vi "экзамен  (SubVI).vi"(6 "N":i32(slide) scale=0.0..10.0, 9 "C":dbl(slide) scale=0.0..10.0, 10 "B":dbl(slide) scale=0.0..10.0, 11 "A":dbl(slide) scale=0.0..10.0) -> ()   [LabVIEW 2012]
panel:
  out "Waveform Graph":dbl[](graph)
  out "Boolean":bool
  out "DC":dbl format="%#_3g"
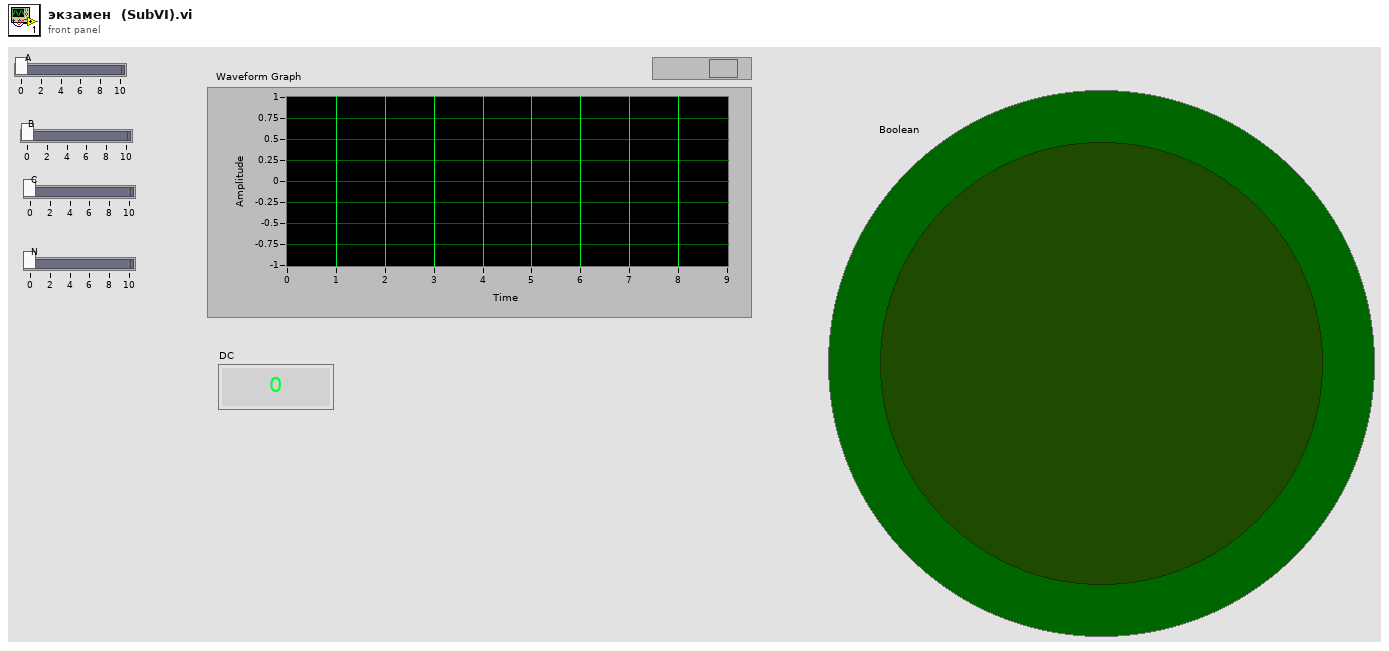
[diagram p1: front panel]
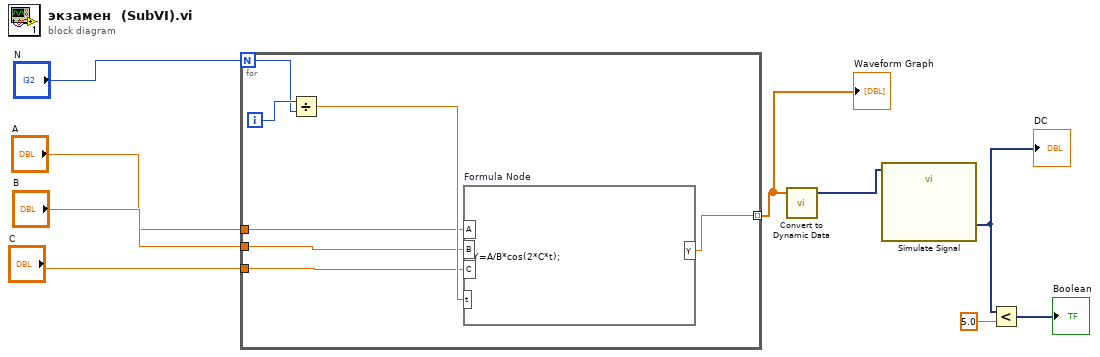
[diagram p0: block diagram]
diagram:
  n1 = for {
    N: "N" -> [w15]
    tunnel: [w13] -> w1 mode=indexing
    tunnel: "A" -> [w12]
    tunnel: "B" -> [w11]
    tunnel: "C" -> [w10]
    i -> [w16]
    n2 = Divide(x=w16, y=w15) -> (x/y=w14:dbl)
    n3 = formula code="Y=A/B*cos(2*C*t);"("B"=w11, "C"=w10, "t"=w14, "A"=w12) -> ("Y"=w13:dbl)
  }
  "Waveform Graph" <- w1
  n4 = call "Convert to Dynamic Data"("Array"=w1) -> ("Dynamic Data Type"=w5:dynamicdata)  [unwired: 3 in]
  n5 = call "Simulate Signal"("Offset"=w5) -> ("DC"=w3:dynamicdata)  [unwired: 13 in, 1 out]
  "DC" <- w3
  n6 = Less?(x=w3, y=5.0) -> (x < y?=→"Boolean":dynamicdata)
